vi "logHardpointActuatorInfo.vi"(8 "error in (no error)":errorcluster, 10 "EventHardpointActuatorInfo":T1, 11 "Communicator in":refnum<class "Communicator.lvclass">) -> (0 "error out":errorcluster, 3 "Communicator out":refnum<class "Communicator.lvclass">)   [LabVIEW 2016, in "M1M3SupportCommunicator.lvlib" / "Communicator.lvclass"]
uses:
  Communicator.lvclass
  DataTypes/Topics/EventHardpointActuatorInfo.ctl
  DataTypes/Topics/Parts/Timestamp.ctl
  DataTypes/Topics/M1M3SupportTopics.lvlib
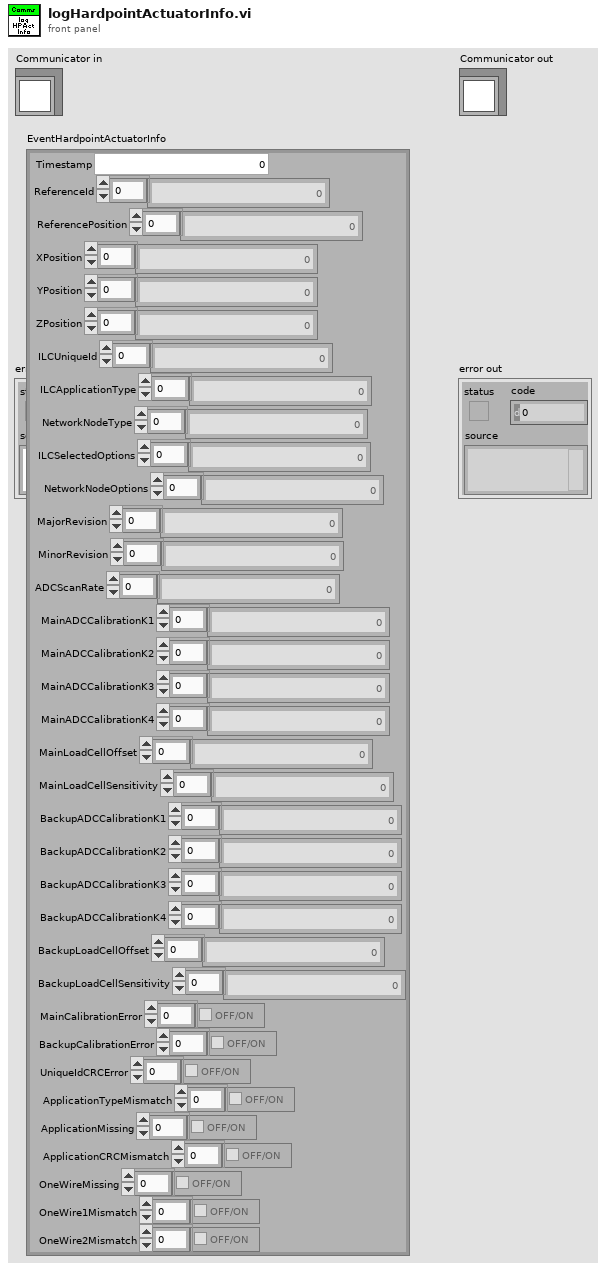
[diagram p1: front panel]
types:
  T1 = typedef "M1M3SupportTopics.lvlib/EventHardpointActuatorInfo.ctl" = cluster{"Timestamp":T2, "ReferenceId":i32[], "ReferencePosition":i32[], "XPosition":sgl[], "YPosition":sgl[], "ZPosition":sgl[], "ILCUniqueId":i64[], "ILCApplicationType":u8[], "NetworkNodeType":u8[], "ILCSelectedOptions":u8[], "NetworkNodeOptions":u8[], "MajorRevision":u8[], "MinorRevision":u8[], "ADCScanRate":u8[], "MainADCCalibrationK1":sgl[], "MainADCCalibrationK2":sgl[], "MainADCCalibrationK3":sgl[], "MainADCCalibrationK4":sgl[], "MainLoadCellOffset":sgl[], "MainLoadCellSensitivity":sgl[], "BackupADCCalibrationK1":sgl[], "BackupADCCalibrationK2":sgl[], "BackupADCCalibrationK3":sgl[], "BackupADCCalibrationK4":sgl[], "BackupLoadCellOffset":sgl[], "BackupLoadCellSensitivity":sgl[], "MainCalibrationError":bool[], "BackupCalibrationError":bool[], "UniqueIdCRCError":bool[], "ApplicationTypeMismatch":bool[], "ApplicationMissing":bool[], "ApplicationCRCMismatch":bool[], "OneWireMissing":bool[], "OneWire1Mismatch":bool[], "OneWire2Mismatch":bool[]}
  T2 = typedef "M1M3SupportTopics.lvlib/Timestamp.ctl" = dbl
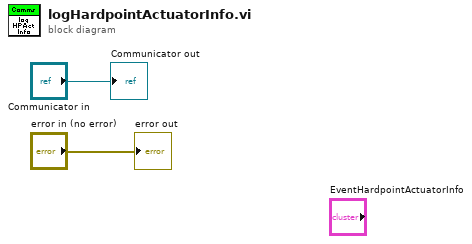
[diagram p0: block diagram]
diagram:
  "error out" <- "error in (no error)"
  "Communicator out" <- "Communicator in"
